vi "Read plugin info.vi"(8 "error in (no error)":errorcluster, 11 "DSFPlugin in":refnum<class "DSFPlugin.lvclass">) -> (0 "error out":errorcluster, 2 "plugin info":T1, 3 "DSFPlugin out":refnum<class "DSFPlugin.lvclass">)   [LabVIEW 2017, in "DSFPlugin.lvclass"]
uses:
  DSFPlugin.lvclass
  Controls/dsf plugin.ctl
  Controls/dsf timing.ctl
  DSFPlugin.lvclass/DSFPlugin.ctl
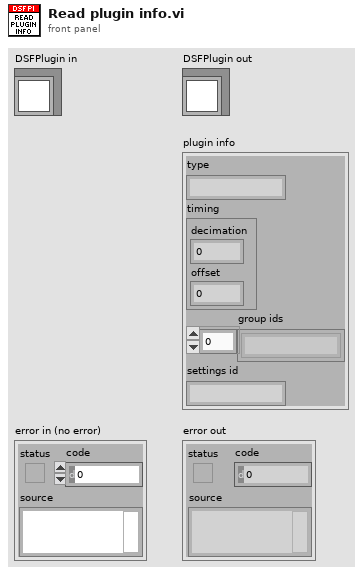
[diagram p1: front panel]
types:
  T1 = typedef "dsf plugin.ctl" = cluster{"type":string, "timing":T2, "group ids":string[], "settings id":string}
  T2 = typedef "dsf timing.ctl" = cluster{"decimation":i32, "offset":i32}
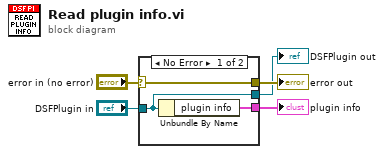
[diagram p0: block diagram]
diagram:
  n1 = case shown="No Error" "error in (no error)" {
    selector: "error in (no error)" -> [w8 w9]
    tunnel: [w8 w9] -> w4
    tunnel: [w7 w10] -> w2
    tunnel: "DSFPlugin in" -> [w7 w10]
    tunnel: [w6 _] -> w1
    frame No Error {
      n2 = Unbundle By Name(w7) -> ("plugin info"=w6:T1)
    }
    frame Error {
    }
  }
  "error out" <- w4
  "DSFPlugin out" <- w2
  "plugin info" <- w1
